vi "ROSServiceProvider.vi"(2 "Response":T2, 3 "ROS":T3={"topic port"=1236, "Node"="/labview", "topic"="/robot/head/command_head_nod", "type"="std_msgs/Bool", "node port"=7000, "error "={"status"=FALSE, "code"=0, "source"=""}, "Direction"=enum."Publisher", "Update (ms)"=1, "FIFO size"=1}) -> ()   [LabVIEW 2016]
doc: "Opens new ports for services, updates services with master, and closes services"
uses:
  SubVIs/_ROSControl.ctl
  SubVIs/_ROSDirection.ctl
  Console/Servers/ServerSubs/MyState.ctl
  _ROSDefinition.vi
panel:
  out "Queue":string
  out "Master Reply":T1(array[cluster])
  out "response":string
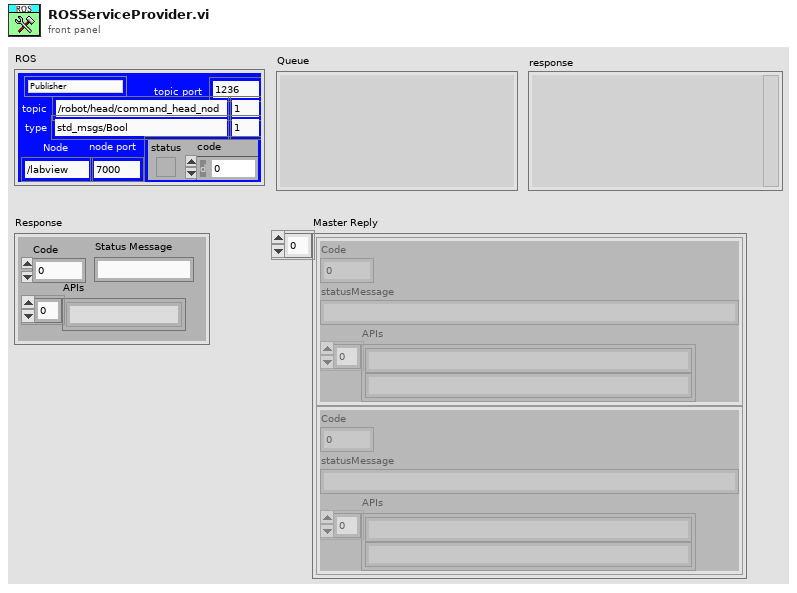
[diagram p1: front panel]
types:
  T1 = cluster{"Code":i8, "statusMessage":string, "APIs":string[]}[]
  T2 = cluster{"Code":i32, "Status Message":string, "APIs":string[]}
  T3 = typedef "_ROSControl.ctl" = cluster{"topic port":u16, "Node":string, "topic":string, "type":string, "node port":u16, "error ":errorcluster, "Direction":T4, "Update (ms)":u16, "FIFO size":u16}
  T4 = typedef "_ROSDirection.ctl" = enum16{"Node", "Publisher", "Subscriber", "ServiceClient", "ServiceProvider"}
  T5 = typedef "MyState.ctl" = enum16{"No Connection", "Registered", "Connected", "Close"}
  T6 = enum16{"Reset Log", "Add Client", "Remove Client", "Add Task"}
  T7 = typedef "ROSLog.ctl" = cluster{"Sent":string, "Reply":string, "MethodName":string, "success":bool, "Dir1":string, "Dir2":string, "Time Stamp":string, "error":errorcluster, "Preamble":string, "Midamble":string, "Postamble":string}
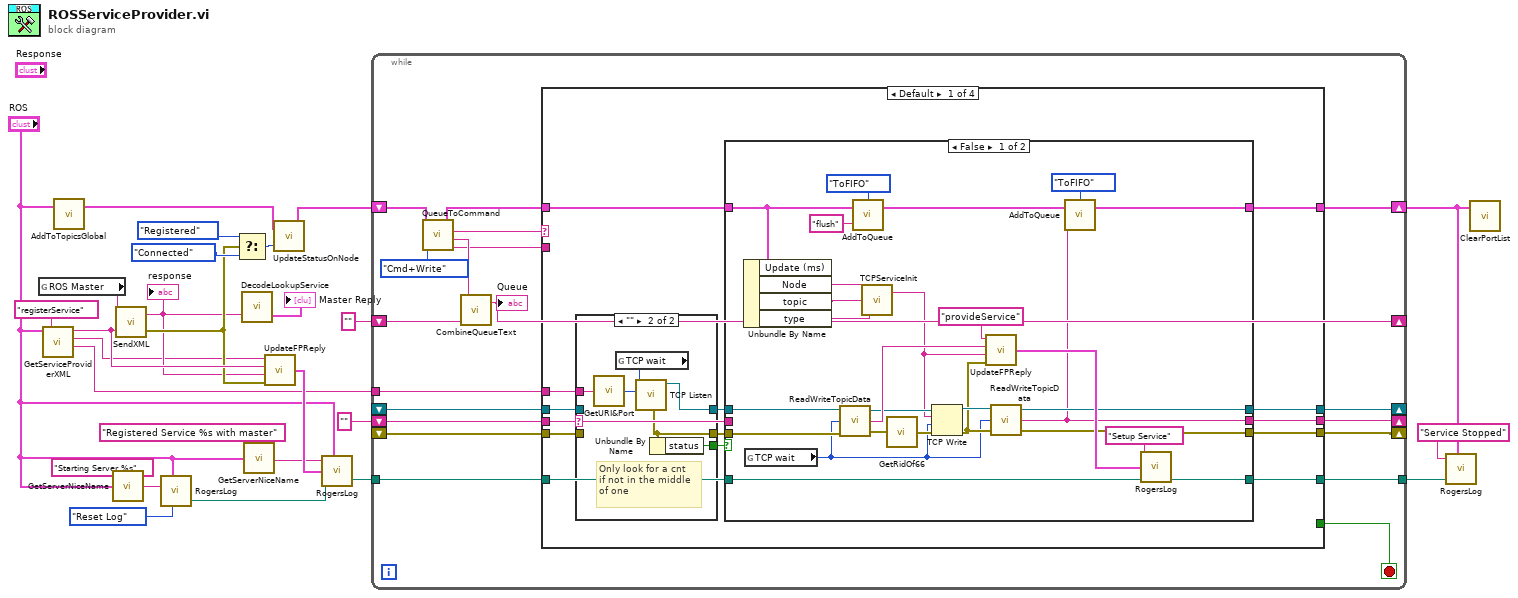
[diagram p0: block diagram]
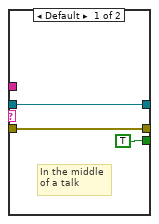
[diagram p2: hidden frame]
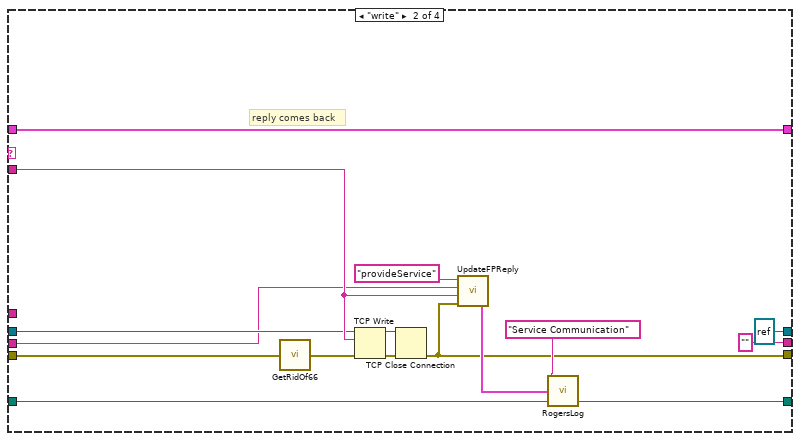
[diagram p4: hidden frame]
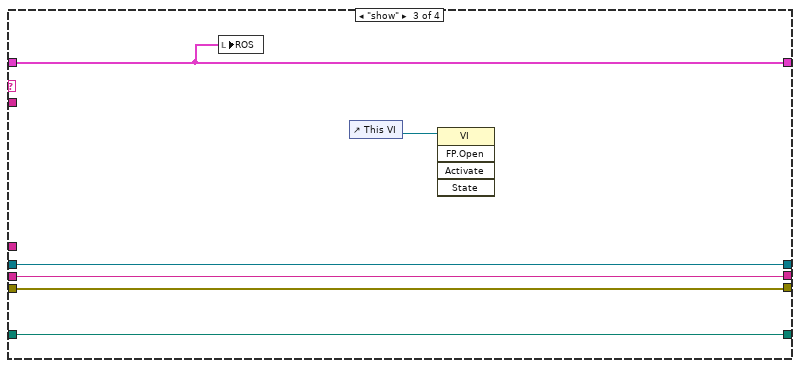
[diagram p5: hidden frame]
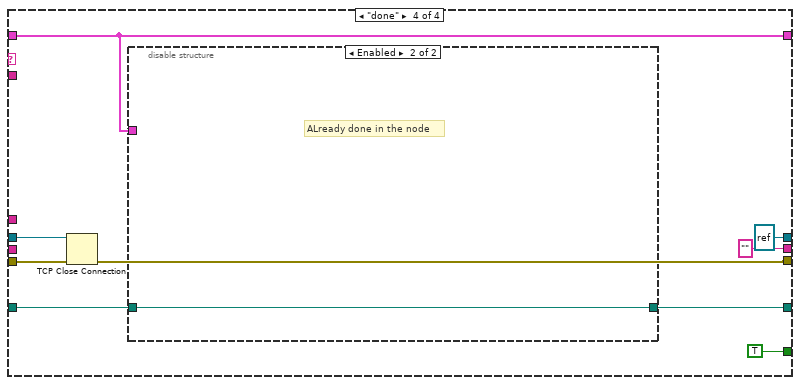
[diagram p6: hidden frame]
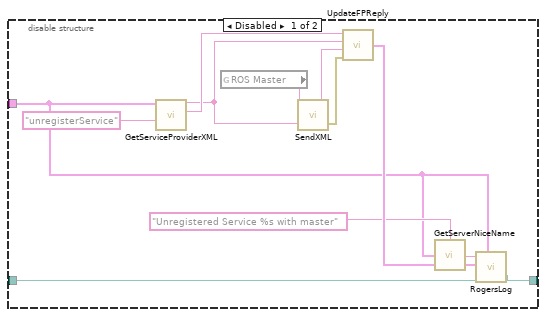
[diagram p7: hidden frame]
diagram:
  n1 = global read "_ROSDefinition.vi" "ROS Master"() -> (w23:string)
  n2 = call "GetServiceProviderXML.vi"("Method Name"="registerService", "ROS"="ROS") -> ("URI"=w6:string, "Method Name"=w9:string, "lookupService"=w24:string)  [unwired: 7 in]
  n3 = call "AddToTopicsGlobal.vi"("ROS in"="ROS") -> ("ROS out"=w3:T3)  [unwired: 2 in]
  n4 = call "GetServerNiceName.vi"("ROS"="ROS", "Text to add"="Starting Server %s") -> ("String"=w26:string)
  n5 = call "SendXML.vi"("Send"=w24, "URI in"=w23) -> ("error out"=w15:errorcluster, "Reply"=w14:string)
  "response" <- w14
  n6 = call "RogersLog.vi"("Text to add"=w26, "ROS"="ROS", "Task"=T6."Reset Log") -> ("LogPath out"=w18:path)  [unwired: 2 in, 1 out]
  n7 = Select(t=MyState."Registered" ("MyState"), s=w15, f=MyState."Connected" ("MyState")) -> (s? t:f=w20:T5)
  n8 = call "DecodeLookupService.vi"("Response"=w14) -> ("Reply"=→"Master Reply":T1)  [unwired: 2 in]
  n9 = call "GetServerNiceName.vi"("ROS"="ROS", "Text to add"="Registered Service %s with master") -> ("String"=w16:string)
  n10 = call "UpdateFPReply.vi"("error in (no error)"=w15, "Reply"=w14, "Sent"=w24, "method"=w9) -> ("Log"=w19:T7)
  n11 = call "UpdateStatusOnNode.vi"("MyState"=w20, "ROS"=w3) -> ("ROS out"=w2:T3)  [unwired: 1 in]
  n12 = call "RogersLog.vi"("Text to add"=w16, "ROS"="ROS", "Log"=w19, "LogPath in"=w18) -> ("LogPath out"=w11:path)  [unwired: 1 in, 1 out]
  n13 = while {
    tunnel: w11 -> [w46]
    tunnel: [w45] -> w10
    shift-right: [w41] -> _
    shift-left: "" ("New List") -> [w42]
    tunnel: w6 -> [w40]
    shift-right: [w36] -> _
    shift-left: _ -> [w33]
    shift-right: [w35] -> _
    shift-left: "" ("data out") -> [w31]
    shift-right: [w34] -> _
    shift-left: _ -> [w32]
    shift-right: [w29] -> w1
    shift-left: w2 -> [w39]
    stop <- w44 stop-if-true
    n14 = call "QueueToCommand.vi"("ROS"=w39, "Check"=enum16{"Cmd+Write", "FIFO", "CMD", "CMD /wait"}."Cmd+Write") -> ("ROS out"=w30:T3, "Command"=w38:string, "Queue log"=w43:string, "data"=w37:string)  [unwired: 1 in]
    n15 = call "CombineQueueText.vi"("Old List"=w42, "Queue In"=w43) -> ("New List"=w41:string)  [unwired: 1 in]
    "Queue" <- w41
    n16 = case shown="Default" w38 {
      tunnel: w30 -> [w59 w104 w118 w131]
      tunnel: w46 -> [w58 w107 w123 w130]
      tunnel: [w57 w106 w123 w129] -> w45
      tunnel: w37 -> [_ w112 _ _]
      tunnel: [w47 w104 w118 w131] -> w29
      tunnel: [_ _ _ TRUE] -> w44
      tunnel: w40 -> [w56 _ _ _]
      tunnel: [w55 refnum<k5> refnum ("connection ID out") w119 refnum<k5> refnum ("connection ID out")] -> w36
      tunnel: [w54 "" ("data out") w120 "" ("data out")] -> w35
      tunnel: [w53 w105 w121 w126] -> w34
      tunnel: w33 -> [w50 w110 w119 w127]
      tunnel: w32 -> [w51 w109 w121 w128]
      tunnel: w31 -> [w52 w108 w120 _]
      frame Default {
        n17 = case shown="\"\"" w52 {
          tunnel: [w63 w65] -> w49
          tunnel: [w62 w68] -> w60
          tunnel: w56 -> [_ w66]
          tunnel: w51 -> [w63 _]
          tunnel: w50 -> [w62 _]
          tunnel: [TRUE w64] -> w48
          frame Default {
            # "In the middle\nof a talk"
          }
          frame "" {
            # "Only look for a cnt\nif not in the middle\nof one"
            n18 = call "GetURI&Port.vi"("URI in"=w66) -> ("Port"=w69:u16)  [unwired: 1 out]
            n19 = global read "_ROSDefinition.vi" "TCP wait"() -> (w67:i32)
            n20 = call "TCP Listen.vi"("timeout ms (wait forever: -1)"=w67, "port"=w69) -> ("error out"=w65:errorcluster, "connection ID"=w68:refnum<k5>)  [unwired: 5 in, 3 out]
            n21 = Unbundle By Name(w65) -> ("status"=w64:bool)
          }
        }
        n22 = case shown="False" w48 {
          tunnel: w60 -> [w96 w100]
          tunnel: w58 -> [w92 w101]
          tunnel: w59 -> [w70 w97]
          tunnel: [w81 w101] -> w57
          tunnel: [w84 w100] -> w55
          tunnel: [w83 w99] -> w54
          tunnel: [w82 w98] -> w53
          tunnel: w52 -> [_ w99]
          tunnel: w49 -> [w80 w98]
          tunnel: [w76 w97] -> w47
          frame False {
            n23 = Unbundle By Name(w70) -> ("Node"=w73:string, "topic"=w72:string, "type"=w74:string)  [unwired: 1 out]
            n24 = global read "_ROSDefinition.vi" "TCP wait"() -> (w79:i32)
            n25 = call "ReadWriteTopicData.vi"("error in (no error)"=w80, "timeout ms (1000)"=w79, "connection ID in"=w96) -> ("error out"=w95:errorcluster, "data out"=w94:string, "connection ID out"=w90:refnum<k5>)
            n26 = call "AddToQueue.vi"("Cmd"="flush", "ROS"=w70, "Type"=enum16{"topic", "node", "ToFIFO", "ToWrite"}."ToFIFO") -> ("ROS out"=w77:T3)  [unwired: 2 in]
            n27 = call "TCPServiceInit.vi"("Type"=w74, "topic"=w72, "callerID"=w73) -> ("TCP ROS Reply"=w71:string)  [unwired: 1 in]
            n28 = call "GetRidOf66.vi"("error in (no error)"=w95) -> ("error out"=w91:errorcluster)
            n29 = TCP Write(connection ID=w90, data in=w71, error in (no error)=w91, 9:w79) -> (connection ID out=w89:refnum<k5>, error out=w88:errorcluster)  [unwired: 1 out]
            n30 = call "UpdateFPReply.vi"("error in (no error)"=w88, "Reply"=w71, "Sent"=w94, "method"="provideService") -> ("Log"=w87:T7)
            n31 = call "ReadWriteTopicData.vi"("error in (no error)"=w88, "timeout ms (1000)"=w79, "connection ID in"=w89) -> ("error out"=w82:errorcluster, "data out"=w83:string, "connection ID out"=w84:refnum<k5>)
            n32 = call "AddToQueue.vi"("Cmd"=w83, "ROS"=w77, "Type"=enum16{"topic", "node", "ToFIFO"}."ToFIFO") -> ("ROS out"=w76:T3)  [unwired: 2 in]
            n33 = call "RogersLog.vi"("Text to add"="Setup Service", "Log"=w87, "LogPath in"=w92) -> ("LogPath out"=w81:path)  [unwired: 2 in, 1 out]
          }
          frame True {
          }
        }
      }
      frame "write" {
        # "reply comes back"
        n34 = call "GetRidOf66.vi"("error in (no error)"=w109) -> ("error out"=w117:errorcluster)
        n35 = TCP Write(connection ID=w110, data in=w112, error in (no error)=w117) -> (connection ID out=w115:refnum<k5>, error out=w116:errorcluster)  [unwired: 1 in, 1 out]
        n36 = TCP Close Connection(connection ID=w115, error in (no error)=w116) -> (error out=w105:errorcluster)  [unwired: 1 in, 1 out]
        n37 = call "UpdateFPReply.vi"("error in (no error)"=w105, "Reply"=w112, "Sent"=w108, "method"="provideService") -> ("Log"=w113:T7)
        n38 = call "RogersLog.vi"("Text to add"="Service Communication", "Log"=w113, "LogPath in"=w107) -> ("LogPath out"=w106:path)  [unwired: 2 in, 1 out]
      }
      frame "show" {
        n39 = local write "ROS"(w118) -> ()
        n40 = control-ref of="This VI"() -> (w122:refnum<vi>)
        n41 = invoke class="VI" method="FP.Open"(reference=w122) -> ()  [unwired: 4 in, 5 out]
      }
      frame "done" {
        n42 = TCP Close Connection(connection ID=w127, error in (no error)=w128) -> (error out=w126:errorcluster)  [unwired: 1 in, 1 out]
        n43 = disable-structure shown="Enabled" {
          disable-tunnel: w131 -> [w136 _]
          disable-tunnel: w130 -> [w134 w145]
          disable-tunnel: [w133 w145] -> w129
          frame Disabled {
            n44 = call "GetServiceProviderXML.vi"("Method Name"="unregisterService", "ROS"=w136) -> ("Method Name"=w141:string, "lookupService"=w140:string)  [unwired: 7 in, 1 out]
            n45 = global read "_ROSDefinition.vi" "ROS Master"() -> (w144:string)
            n46 = call "SendXML.vi"("Send"=w140, "URI in"=w144) -> ("error out"=w142:errorcluster, "Reply"=w139:string)
            n47 = call "UpdateFPReply.vi"("error in (no error)"=w142, "Reply"=w139, "Sent"=w140, "method"=w141) -> ("Log"=w138:T7)
            n48 = call "GetServerNiceName.vi"("ROS"=w136, "Text to add"="Unregistered Service %s with master") -> ("String"=w135:string)
            n49 = call "RogersLog.vi"("Text to add"=w135, "ROS"=w136, "Log"=w138, "LogPath in"=w134) -> ("LogPath out"=w133:path)  [unwired: 1 in, 1 out]
          }
          frame Enabled {
            # "ALready done in the node"
          }
        }
      }
    }
  }
  n50 = call "RogersLog.vi"("Text to add"="Service Stopped", "ROS"=w1, "LogPath in"=w10) -> ()  [unwired: 2 in, 2 out]
  n51 = call "ClearPortList.vi"("ROS"=w1) -> ()  [unwired: 2 in]
